vi "Force_command_IHS.vi"(11 "Data In":T1={"Core"={"Current VI Reference"=refnum, "Close Panel on Exit?"=FALSE, "Start Timestmap"="", "Status His"="", "Active"=FALSE, "Exit"=FALSE, "Assignment structure"=""}, "Sample ID"="", "Cam"={"Cam"="", "Connected"=FALSE, "Sim Image"=FALSE, "Save pictures"=FALSE}, "UR"={"PC_IP"="192.168.0.15", "Remote port"=30002, "UR_IP"="192.168.0.10", "connection ID"=refnum, "Connected"=FALSE, "Sim UR signal"=FALSE, "UR Ready"=FALSE, "Ready fail"=0.0}, "Sample data"={"Insects taken from current picture"=0, "Number of insects in pick-up area"=0, "Object data"={"Object CoM X"=0.0, "Object CoM Y"=0.0, "Corrected Object orientation"=0.0, "Object length"=0.0, "Z, Height"=0.0}, "Raw Particle Measurements"=[], "Insect-data-array"=[], "Sorted Particle Measurements"=[], "Insects to pick this round"=0, "Picking array"=[], "Pixels Measurements"=[], "Tool1 to pick"=0}, "Images"={"Image"=refnum, "Image Timestamp"="", "Boarder Image"=refnum, "Vision A. Image"=refnum}, "Reshake"=0, "Settings"={"Number to try and pick"=8, "Last few"=4, "Z_Zero"=0.0, "Tool switch size"=2.0, "X-Zero"=-35.0, "Y-Zero"=406.0, "Small or XL"=12.0, "Tool1-Height"=12.0, "Tool2-Height"=12.0, "Ignore small"=12.0, "Time to Whait"=25.0}, "Assignment"={"Executing Assignment"="", "Task"="", "Tool"="", "Specimen to pick"=0, "GO"=FALSE}, "Return reason"=""} {"Sample data"."Object data"."Z, Height" format="%#_13g"}) -> (1 "Command type":enum16{"Default", "Right", "Left"}(ring), 2 "Canceled":bool, 3 "Data Out":T1={"Core"={"Current VI Reference"=refnum, "Close Panel on Exit?"=FALSE, "Start Timestmap"="", "Status His"="", "Active"=FALSE, "Exit"=FALSE, "Assignment structure"=""}, "Sample ID"="", "Cam"={"Cam"="", "Connected"=FALSE, "Sim Image"=FALSE, "Save pictures"=FALSE}, "UR"={"PC_IP"="192.168.0.15", "Remote port"=30002, "UR_IP"="192.168.0.10", "connection ID"=refnum, "Connected"=FALSE, "Sim UR signal"=FALSE, "UR Ready"=FALSE, "Ready fail"=0.0}, "Sample data"={"Insects taken from current picture"=0, "Number of insects in pick-up area"=0, "Object data"={"Object CoM X"=0.0, "Object CoM Y"=0.0, "Corrected Object orientation"=0.0, "Object length"=0.0, "Z, Height"=0.0}, "Raw Particle Measurements"=[], "Insect-data-array"=[], "Sorted Particle Measurements"=[], "Insects to pick this round"=0, "Picking array"=[], "Pixels Measurements"=[], "Tool1 to pick"=0}, "Images"={"Image"=refnum, "Image Timestamp"="", "Boarder Image"=refnum, "Vision A. Image"=refnum}, "Reshake"=0, "Settings"={"Number to try and pick"=8, "Last few"=4, "Z_Zero"=0.1, "Tool switch size"=2.0, "X-Zero"=-35.0, "Y-Zero"=406.0, "Small or XL"=12.0, "Tool1-Height"=12.0, "Tool2-Height"=12.0, "Ignore small"=12.0, "Time to Whait"=25.0}, "Assignment"={"Executing Assignment"="", "Task"="", "Tool"="", "Specimen to pick"=0, "GO"=FALSE}, "Return reason"=""} {"Sample data"."Object data"."Z, Height" format="%#_13g"})   [LabVIEW 2024]
uses:
  SRS/controls/IHS_JKI.ctl
  <vilib>/userDefined/High Color/IMAQdx.ctl
  <vilib>/vision/Image Controls.llb/IMAQ Image.ctl
panel:
  in  "Left":T4
  in  "Right":cluster{"Specimen to pick":i32}
  out "Sample data.Insect-data-array":string[][](array[string])
  in  "Cancel Button":bool
  in  "OK Button":bool
  # "UR Task list:\n1 = take pic.\n2 = take pic. No light.\n3-6 = Shake.\n7 = Sample for Sta. Bio with Tool1.\n8 = Sample for Sta. Bio with Tool2.\n9 = Tool3.\n10 = Move with selected Tool to specified pos.\n14 = Sample for XL Bio. with Tool1.\n16 = Sample for XL Bio. with Tool2.\n55 = Reset UR"
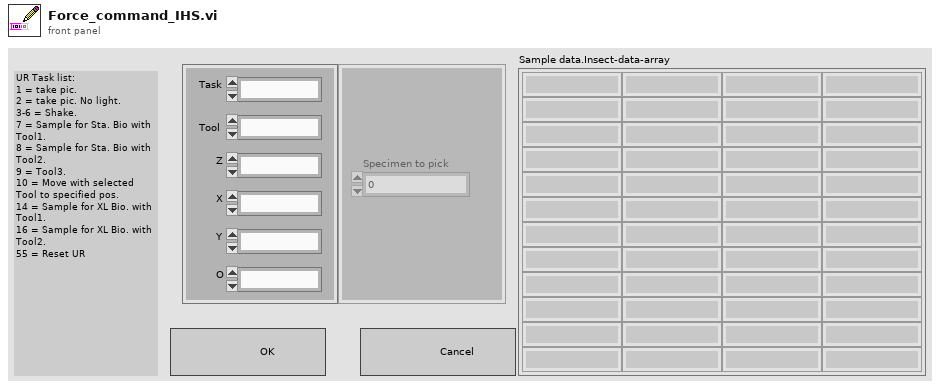
[diagram p1: front panel]
types:
  T1 = typedef "IHS_JKI.ctl" = cluster{"Core":cluster{"Current VI Reference":refnum<vi>, "Close Panel on Exit?":bool, "Start Timestmap":string, "Status His":string, "Active":bool, "Exit":bool, "Assignment structure":string}, "Sample ID":string, "Cam":cluster{"Cam":T2, "Connected":bool, "Sim Image":bool, "Save pictures":bool}, "UR":cluster{"PC_IP":string, "Remote port":u16, "UR_IP":string, "connection ID":refnum<k5>, "Connected":bool, "Sim UR signal":bool, "UR Ready":bool, "Ready fail":dbl}, "Sample data":cluster{"Insects taken from current picture":i32, "Number of insects in pick-up area":i32, "Object data":cluster{"Object CoM X":dbl, "Object CoM Y":dbl, "Corrected Object orientation":dbl, "Object length":dbl, "Z, Height":dbl}, "Raw Particle Measurements":dbl[][], "Insect-data-array":string[][], "Sorted Particle Measurements":dbl[][], "Insects to pick this round":i32, "Picking array":dbl[][], "Pixels Measurements":dbl[][], "Tool1 to pick":i32}, "Images":cluster{"Image":T3, "Image Timestamp":string, "Boarder Image":T3, "Vision A. Image":T3}, "Reshake":i32, "Settings":cluster{"Number to try and pick":i32, "Last few":i32, "Z_Zero":dbl, "Tool switch size":dbl, "X-Zero":dbl, "Y-Zero":dbl, "Small or XL":dbl, "Tool1-Height":dbl, "Tool2-Height":dbl, "Ignore small":dbl, "Time to Whait":dbl}, "Assignment":cluster{"Executing Assignment":string, "Task":string, "Tool":string, "Specimen to pick":i32, "GO":bool}, "Return reason":string}
  T2 = typedef "IMAQdx.ctl" = refnum<k21>
  T3 = typedef "IMAQ Image.ctl" = refnum<image>
  T4 = cluster{"Task":i32, "Tool":i32, "Y":dbl, "X":dbl, "Z":dbl, "O":dbl}
  T5 = enum8{"Enabled", "Disabled", "Disabled and Grayed Out"}
  T6 = cluster{"Number to try and pick":i32, "Last few":i32, "Z_Zero":dbl, "Tool switch size":dbl, "X-Zero":dbl, "Y-Zero":dbl, "Small or XL":dbl, "Tool1-Height":dbl, "Tool2-Height":dbl, "Ignore small":dbl, "Time to Whait":dbl}
  T7 = cluster{"Executing Assignment":string, "Task":string, "Tool":string, "Specimen to pick":i32, "GO":bool}
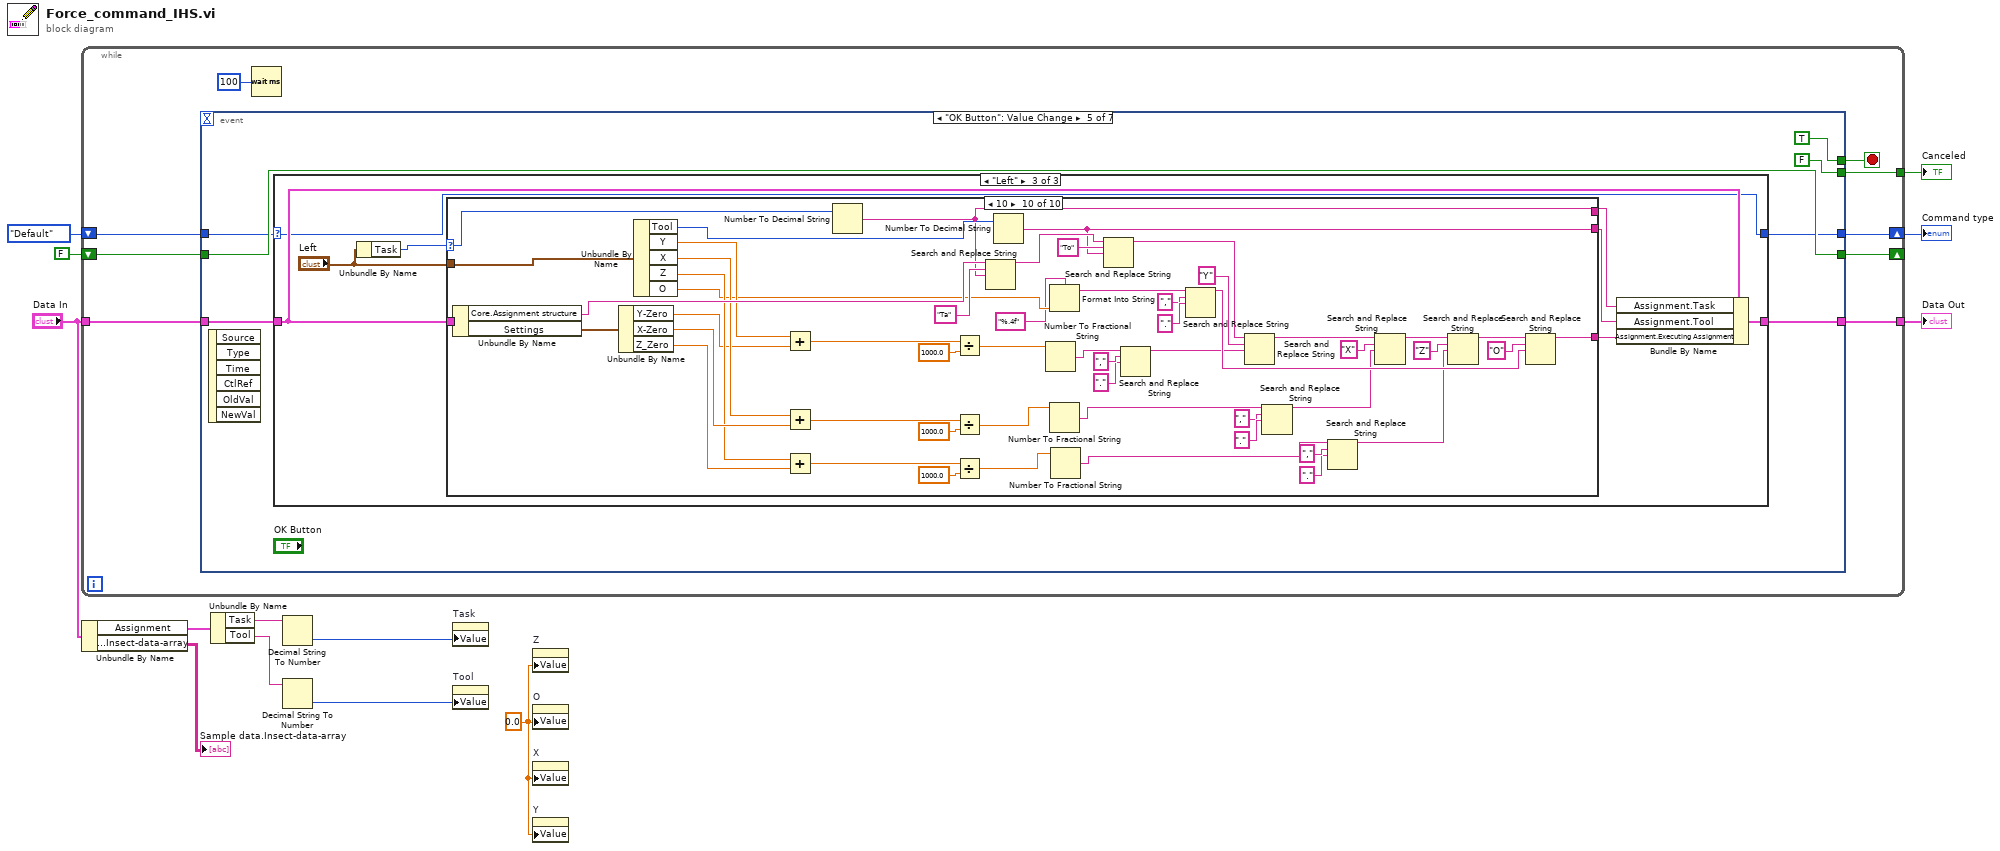
[diagram p0: block diagram]
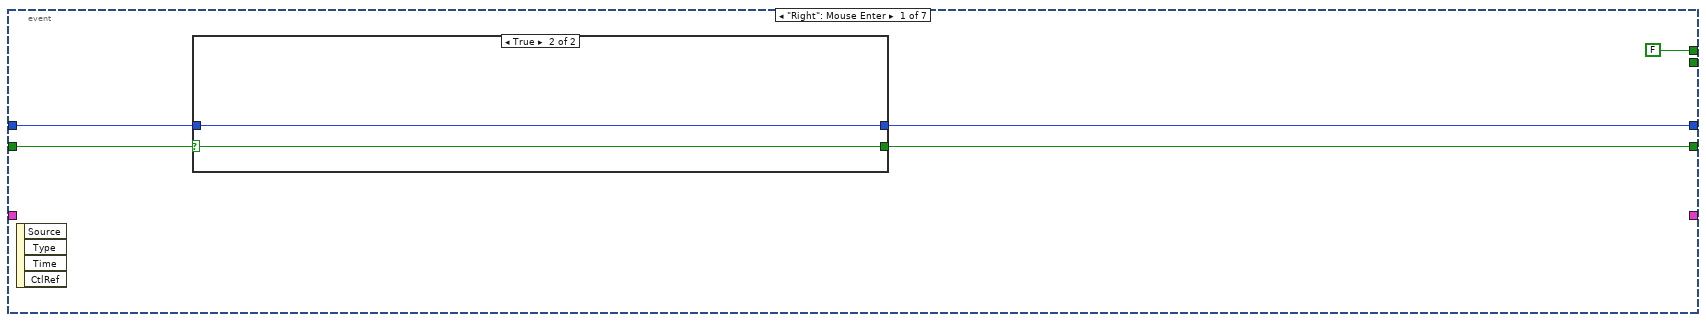
[diagram p2: hidden frame]
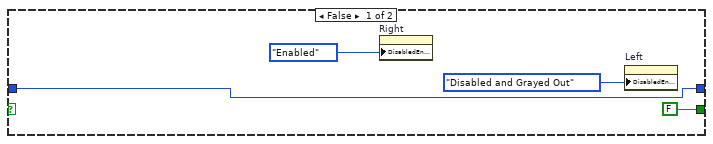
[diagram p3: hidden frame]
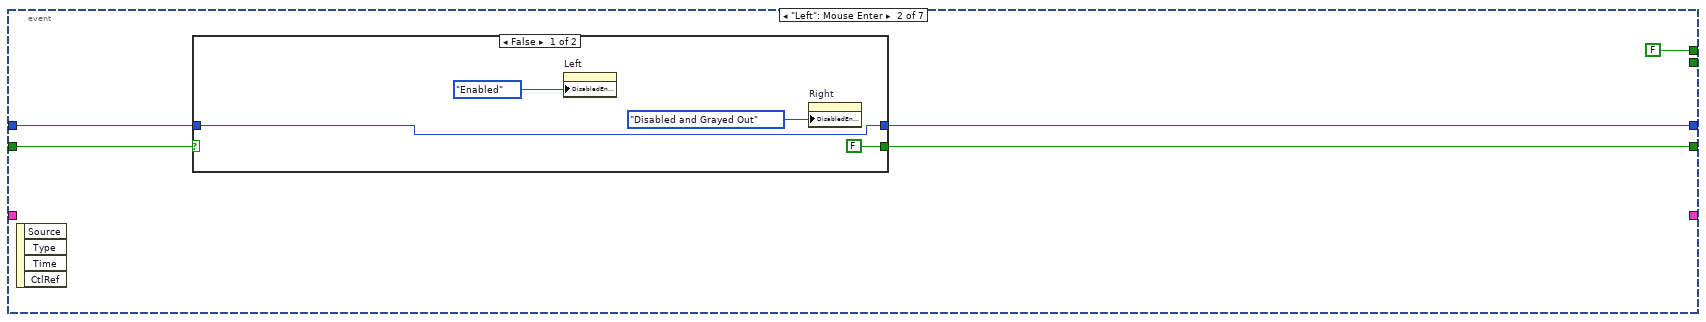
[diagram p4: hidden frame]
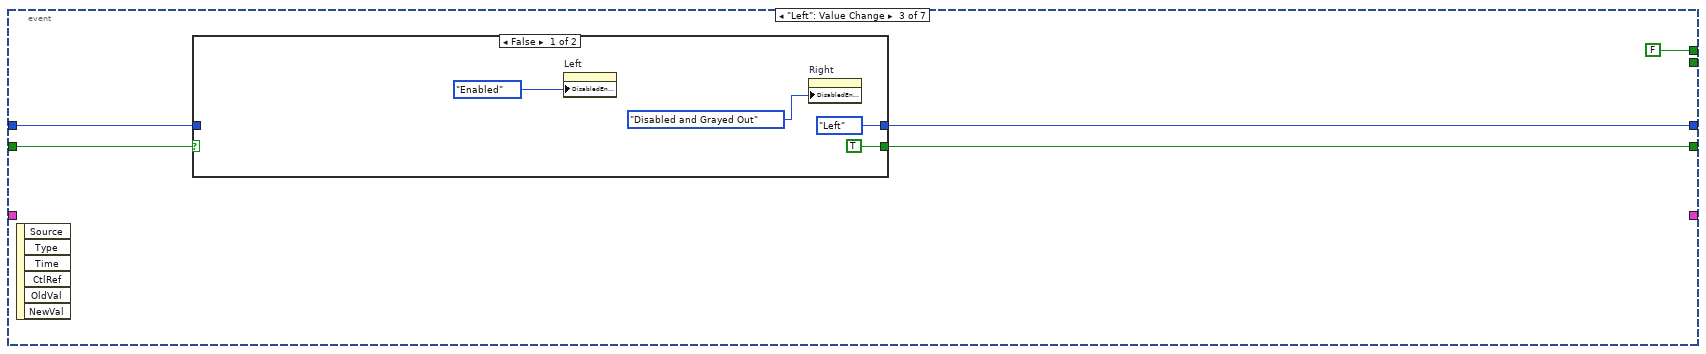
[diagram p6: hidden frame]
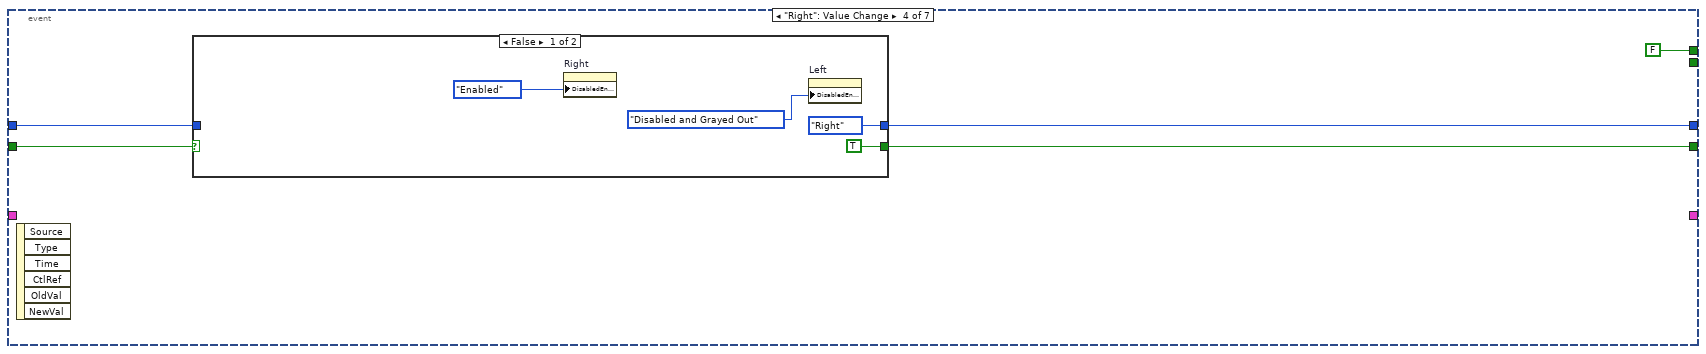
[diagram p8: hidden frame]
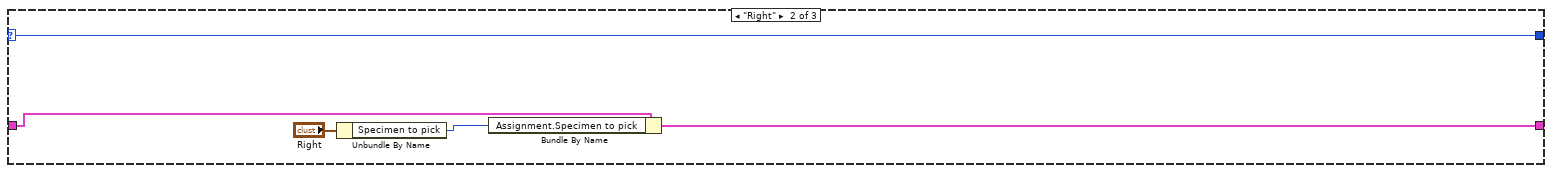
[diagram p11: hidden frame]
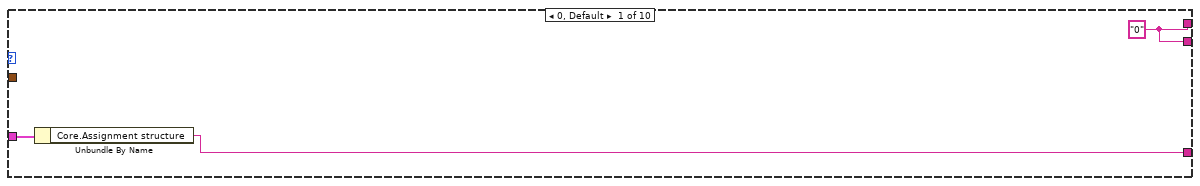
[diagram p12: hidden frame]
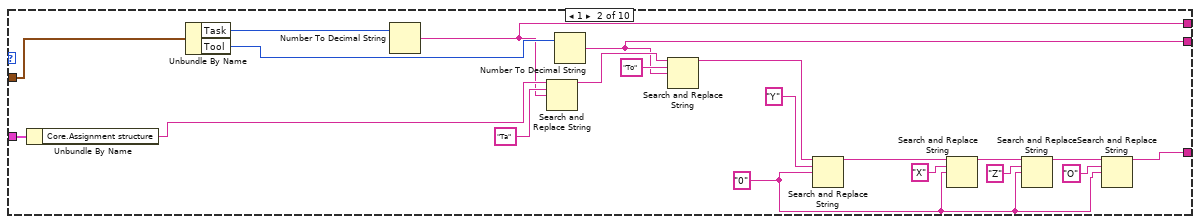
[diagram p13: hidden frame]
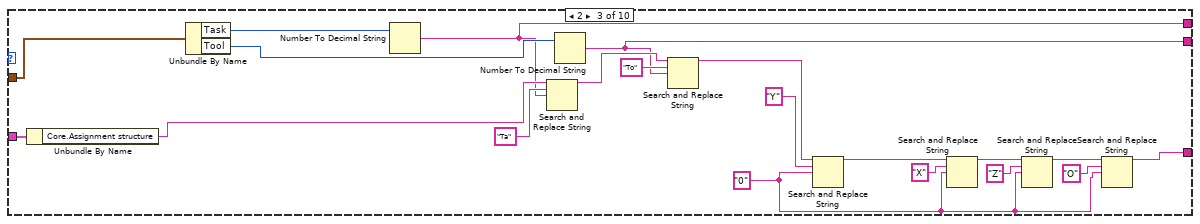
[diagram p14: hidden frame]
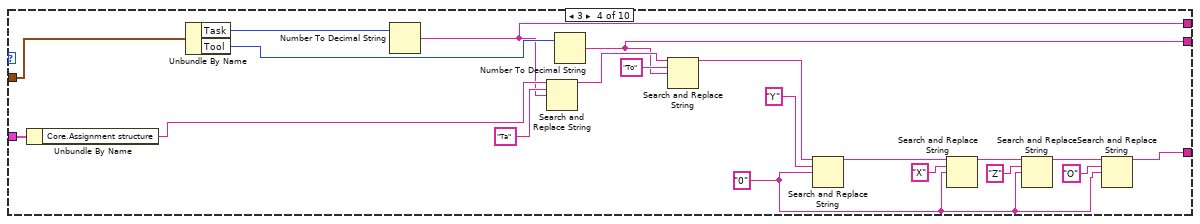
[diagram p15: hidden frame]
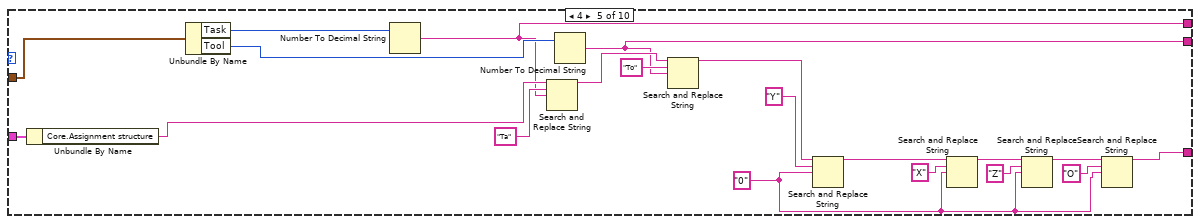
[diagram p16: hidden frame]
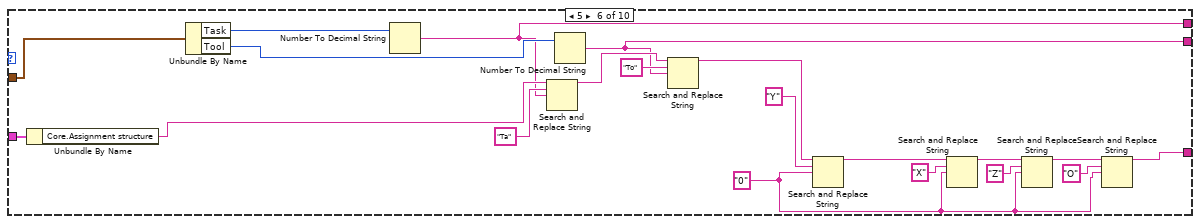
[diagram p17: hidden frame]
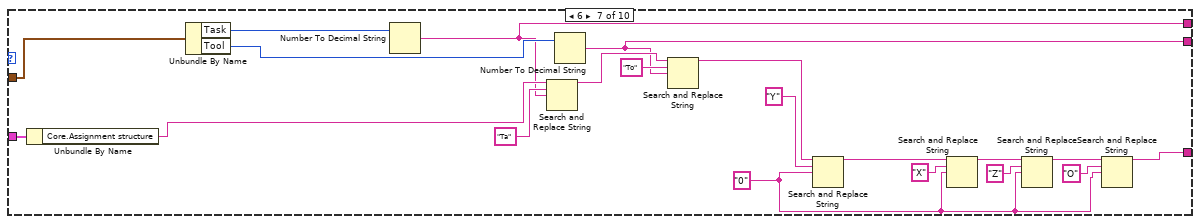
[diagram p18: hidden frame]
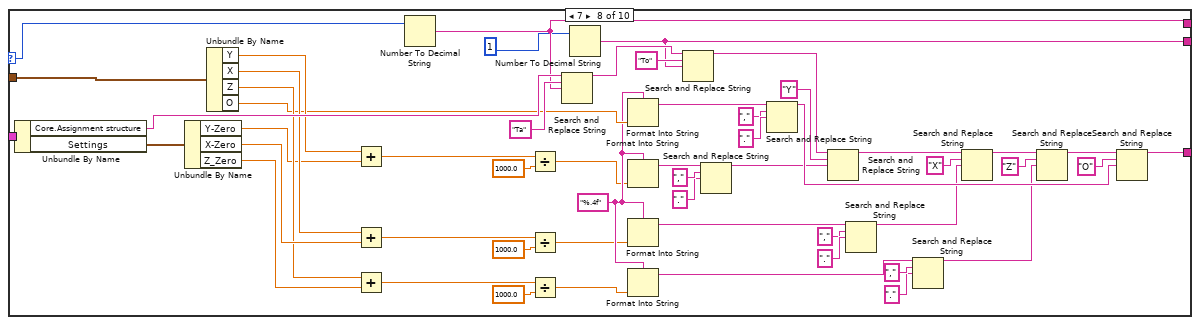
[diagram p19: hidden frame]
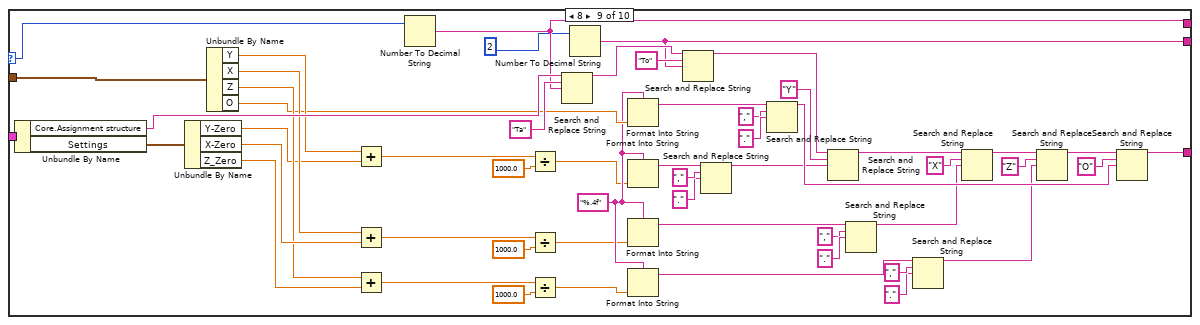
[diagram p20: hidden frame]
diagram:
  w1 = 0.0 ("Value")
  n1 = while {
    shift-right: [w20] -> _
    shift-left: FALSE -> [w21]
    shift-right: [w19] -> w5
    shift-left: enum16{"Default", "Right", "Left"}."Default" -> [w18]
    tunnel: "Data In" -> [w17]
    tunnel: [w16] -> w6
    tunnel: [w15] -> w4
    stop <- w14 stop-if-true
    n2 = event shown="[4] \"OK Button\": Value Change" {
      selector: _ -> [_ _ _ _ _ _ _]
      dyn-events: _ -> [_ _ _ _ _ _ _]
      timeout: _ -> [_ _ _ _ _ _ _]
      tunnel: [w27 w38 w47 w60 w72 w373 _] -> w20
      tunnel: [w26 w37 w49 w59 w68 enum16{"Default", "Right", "Left"}."Default" enum16{"Default", "Right", "Left"}."Default"] -> w19
      tunnel: w21 -> [w25 w36 w48 w58 w72 w373 _]
      tunnel: w18 -> [w24 w35 w46 w57 w69 _ _]
      tunnel: w17 -> [_ _ _ _ w73 w374 w378]
      tunnel: [_ _ _ _ FALSE TRUE TRUE] -> w16
      tunnel: [_ _ _ _ w70 w374 w378] -> w15
      tunnel: [FALSE FALSE FALSE FALSE TRUE TRUE TRUE] -> w14
      event "Right": Mouse Enter {
        n3 = event-data() -> ()  [unwired: 1 in, 4 out]
        n4 = case shown="True" w25 {
          selector: w25 -> [_ w33]
          tunnel: [FALSE w33] -> w27
          tunnel: [w28 w32] -> w26
          tunnel: w24 -> [w28 w32]
          frame False {
            n5 = property on="Right" class="Clust (strict)"("DisabledEnum"=T5."Enabled" ("Disabled")) -> ()  [unwired: 2 in, 2 out]
            n6 = property on="Left" class="Clust (strict)"("DisabledEnum"=T5."Disabled and Grayed Out" ("Disabled")) -> ()  [unwired: 2 in, 2 out]
          }
          frame True {
          }
        }
      }
      event "Left": Mouse Enter {
        n7 = event-data() -> ()  [unwired: 1 in, 4 out]
        n8 = case shown="False" w36 {
          selector: w36 -> [_ w44]
          tunnel: [FALSE w44] -> w38
          tunnel: [w39 w43] -> w37
          tunnel: w35 -> [w39 w43]
          frame False {
            n9 = property on="Left" class="Clust (strict)"("DisabledEnum"=T5."Enabled" ("Disabled")) -> ()  [unwired: 2 in, 2 out]
            n10 = property on="Right" class="Clust (strict)"("DisabledEnum"=T5."Disabled and Grayed Out" ("Disabled")) -> ()  [unwired: 2 in, 2 out]
          }
          frame True {
          }
        }
      }
      event "Left": Value Change {
        n11 = event-data() -> ()  [unwired: 1 in, 6 out]
        n12 = case shown="False" w48 {
          selector: w48 -> [_ w55]
          tunnel: [enum16{"Default", "Right", "Left"}."Left" w54] -> w49
          tunnel: [TRUE w55] -> w47
          tunnel: w46 -> [_ w54]
          frame False {
            n13 = property on="Left" class="Clust (strict)"("DisabledEnum"=T5."Enabled" ("Disabled")) -> ()  [unwired: 2 in, 2 out]
            n14 = property on="Right" class="Clust (strict)"("DisabledEnum"=T5."Disabled and Grayed Out" ("Disabled")) -> ()  [unwired: 2 in, 2 out]
          }
          frame True {
          }
        }
      }
      event "Right": Value Change {
        n15 = event-data() -> ()  [unwired: 1 in, 6 out]
        n16 = case shown="False" w58 {
          selector: w58 -> [_ w66]
          tunnel: [TRUE w66] -> w60
          tunnel: [enum16{"Default", "Right", "Left"}."Right" w65] -> w59
          tunnel: w57 -> [_ w65]
          frame False {
            n17 = property on="Right" class="Clust (strict)"("DisabledEnum"=T5."Enabled" ("Disabled")) -> ()  [unwired: 2 in, 2 out]
            n18 = property on="Left" class="Clust (strict)"("DisabledEnum"=T5."Disabled and Grayed Out" ("Disabled")) -> ()  [unwired: 2 in, 2 out]
          }
          frame True {
          }
        }
      }
      event "OK Button": Value Change {
        n19 = event-data() -> ()  [unwired: 1 in, 6 out]
        n20 = case shown="\"Left\"" w69 {
          selector: w69 -> [w74 w77 w84]
          tunnel: w73 -> [w75 w80 w88]
          tunnel: [w75 w79 w85] -> w70
          tunnel: [w74 w77 w84] -> w68
          frame "Default", Default {
          }
          frame "Right" {
            n21 = Unbundle By Name("Right") -> ("Specimen to pick"=w78:i32)
            n22 = Bundle By Name(cluster=w80, "Assignment.Specimen to pick"=w78) -> (w79:T1)
          }
          frame "Left" {
            n23 = Unbundle By Name("Left") -> ("Task"=w81:i32)
            n24 = case shown="10" w81 {
              selector: w81 -> [_ _ _ _ _ _ _ w214 w267 w325]
              tunnel: w88 -> [w91 w99 w119 w139 w159 w179 w199 w264 w317 w370]
              tunnel: [w89 w94 w114 w134 w154 w174 w194 w213 w266 w324] -> w87
              tunnel: [w89 w93 w113 w133 w153 w173 w193 w253 w306 w358] -> w86
              tunnel: "Left" -> [_ w97 w117 w137 w157 w177 w197 w252 w305 w357]
              tunnel: [w90 w95 w115 w135 w155 w175 w195 w243 w296 w348] -> w83
              frame 0, Default {
                w89 = "0"
                n25 = Unbundle By Name(w91) -> ("Core.Assignment structure"=w90:string)
              }
              frame 1 {
                w92 = "0" ("replace string (\"\")")
                n26 = Unbundle By Name(w99) -> ("Core.Assignment structure"=w98:string)
                n27 = Unbundle By Name(w97) -> ("Task"=w96:i32, "Tool"=w111:i32)
                n28 = Number To Decimal String(number=w96) -> (decimal integer string=w94:string)  [unwired: 1 in]
                n29 = Search and Replace String(input string=w98, search string="Ta", replace string=w94) -> (result string=w110:string)  [unwired: 5 in, 3 out]
                n30 = Number To Decimal String(number=w111) -> (decimal integer string=w93:string)  [unwired: 1 in]
                n31 = Search and Replace String(input string=w110, search string="To", replace string=w93) -> (result string=w109:string)  [unwired: 5 in, 3 out]
                n32 = Search and Replace String(input string=w109, search string="Y", replace string=w92) -> (result string=w108:string)  [unwired: 5 in, 3 out]
                n33 = Search and Replace String(input string=w108, search string="X", replace string=w92) -> (result string=w107:string)  [unwired: 5 in, 3 out]
                n34 = Search and Replace String(input string=w107, search string="Z", replace string=w92) -> (result string=w101:string)  [unwired: 5 in, 3 out]
                n35 = Search and Replace String(input string=w101, search string="O", replace string=w92) -> (result string=w95:string)  [unwired: 5 in, 3 out]
              }
              frame 2 {
                w112 = "0" ("replace string (\"\")")
                n36 = Unbundle By Name(w119) -> ("Core.Assignment structure"=w118:string)
                n37 = Unbundle By Name(w117) -> ("Task"=w116:i32, "Tool"=w131:i32)
                n38 = Number To Decimal String(number=w116) -> (decimal integer string=w114:string)  [unwired: 1 in]
                n39 = Search and Replace String(input string=w118, search string="Ta", replace string=w114) -> (result string=w130:string)  [unwired: 5 in, 3 out]
                n40 = Number To Decimal String(number=w131) -> (decimal integer string=w113:string)  [unwired: 1 in]
                n41 = Search and Replace String(input string=w130, search string="To", replace string=w113) -> (result string=w129:string)  [unwired: 5 in, 3 out]
                n42 = Search and Replace String(input string=w129, search string="Y", replace string=w112) -> (result string=w128:string)  [unwired: 5 in, 3 out]
                n43 = Search and Replace String(input string=w128, search string="X", replace string=w112) -> (result string=w127:string)  [unwired: 5 in, 3 out]
                n44 = Search and Replace String(input string=w127, search string="Z", replace string=w112) -> (result string=w121:string)  [unwired: 5 in, 3 out]
                n45 = Search and Replace String(input string=w121, search string="O", replace string=w112) -> (result string=w115:string)  [unwired: 5 in, 3 out]
              }
              frame 3 {
                w132 = "0" ("replace string (\"\")")
                n46 = Unbundle By Name(w139) -> ("Core.Assignment structure"=w138:string)
                n47 = Unbundle By Name(w137) -> ("Task"=w136:i32, "Tool"=w151:i32)
                n48 = Number To Decimal String(number=w136) -> (decimal integer string=w134:string)  [unwired: 1 in]
                n49 = Search and Replace String(input string=w138, search string="Ta", replace string=w134) -> (result string=w150:string)  [unwired: 5 in, 3 out]
                n50 = Number To Decimal String(number=w151) -> (decimal integer string=w133:string)  [unwired: 1 in]
                n51 = Search and Replace String(input string=w150, search string="To", replace string=w133) -> (result string=w149:string)  [unwired: 5 in, 3 out]
                n52 = Search and Replace String(input string=w149, search string="Y", replace string=w132) -> (result string=w148:string)  [unwired: 5 in, 3 out]
                n53 = Search and Replace String(input string=w148, search string="X", replace string=w132) -> (result string=w147:string)  [unwired: 5 in, 3 out]
                n54 = Search and Replace String(input string=w147, search string="Z", replace string=w132) -> (result string=w141:string)  [unwired: 5 in, 3 out]
                n55 = Search and Replace String(input string=w141, search string="O", replace string=w132) -> (result string=w135:string)  [unwired: 5 in, 3 out]
              }
              frame 4 {
                w152 = "0" ("replace string (\"\")")
                n56 = Unbundle By Name(w159) -> ("Core.Assignment structure"=w158:string)
                n57 = Unbundle By Name(w157) -> ("Task"=w156:i32, "Tool"=w171:i32)
                n58 = Number To Decimal String(number=w156) -> (decimal integer string=w154:string)  [unwired: 1 in]
                n59 = Search and Replace String(input string=w158, search string="Ta", replace string=w154) -> (result string=w170:string)  [unwired: 5 in, 3 out]
                n60 = Number To Decimal String(number=w171) -> (decimal integer string=w153:string)  [unwired: 1 in]
                n61 = Search and Replace String(input string=w170, search string="To", replace string=w153) -> (result string=w169:string)  [unwired: 5 in, 3 out]
                n62 = Search and Replace String(input string=w169, search string="Y", replace string=w152) -> (result string=w168:string)  [unwired: 5 in, 3 out]
                n63 = Search and Replace String(input string=w168, search string="X", replace string=w152) -> (result string=w167:string)  [unwired: 5 in, 3 out]
                n64 = Search and Replace String(input string=w167, search string="Z", replace string=w152) -> (result string=w161:string)  [unwired: 5 in, 3 out]
                n65 = Search and Replace String(input string=w161, search string="O", replace string=w152) -> (result string=w155:string)  [unwired: 5 in, 3 out]
              }
              frame 5 {
                w172 = "0" ("replace string (\"\")")
                n66 = Unbundle By Name(w179) -> ("Core.Assignment structure"=w178:string)
                n67 = Unbundle By Name(w177) -> ("Task"=w176:i32, "Tool"=w191:i32)
                n68 = Number To Decimal String(number=w176) -> (decimal integer string=w174:string)  [unwired: 1 in]
                n69 = Search and Replace String(input string=w178, search string="Ta", replace string=w174) -> (result string=w190:string)  [unwired: 5 in, 3 out]
                n70 = Number To Decimal String(number=w191) -> (decimal integer string=w173:string)  [unwired: 1 in]
                n71 = Search and Replace String(input string=w190, search string="To", replace string=w173) -> (result string=w189:string)  [unwired: 5 in, 3 out]
                n72 = Search and Replace String(input string=w189, search string="Y", replace string=w172) -> (result string=w188:string)  [unwired: 5 in, 3 out]
                n73 = Search and Replace String(input string=w188, search string="X", replace string=w172) -> (result string=w187:string)  [unwired: 5 in, 3 out]
                n74 = Search and Replace String(input string=w187, search string="Z", replace string=w172) -> (result string=w181:string)  [unwired: 5 in, 3 out]
                n75 = Search and Replace String(input string=w181, search string="O", replace string=w172) -> (result string=w175:string)  [unwired: 5 in, 3 out]
              }
              frame 6 {
                w192 = "0" ("replace string (\"\")")
                n76 = Unbundle By Name(w199) -> ("Core.Assignment structure"=w198:string)
                n77 = Unbundle By Name(w197) -> ("Task"=w196:i32, "Tool"=w211:i32)
                n78 = Number To Decimal String(number=w196) -> (decimal integer string=w194:string)  [unwired: 1 in]
                n79 = Search and Replace String(input string=w198, search string="Ta", replace string=w194) -> (result string=w210:string)  [unwired: 5 in, 3 out]
                n80 = Number To Decimal String(number=w211) -> (decimal integer string=w193:string)  [unwired: 1 in]
                n81 = Search and Replace String(input string=w210, search string="To", replace string=w193) -> (result string=w209:string)  [unwired: 5 in, 3 out]
                n82 = Search and Replace String(input string=w209, search string="Y", replace string=w192) -> (result string=w208:string)  [unwired: 5 in, 3 out]
                n83 = Search and Replace String(input string=w208, search string="X", replace string=w192) -> (result string=w207:string)  [unwired: 5 in, 3 out]
                n84 = Search and Replace String(input string=w207, search string="Z", replace string=w192) -> (result string=w201:string)  [unwired: 5 in, 3 out]
                n85 = Search and Replace String(input string=w201, search string="O", replace string=w192) -> (result string=w195:string)  [unwired: 5 in, 3 out]
              }
              frame 7 {
                w226 = "%.4f" ("format string")
                n86 = Unbundle By Name(w264) -> ("Core.Assignment structure"=w263:string, "Settings"=w251:T6)
                n87 = Unbundle By Name(w251) -> ("Y-Zero"=w245:dbl, "X-Zero"=w248:dbl, "Z_Zero"=w246:dbl)
                n88 = Unbundle By Name(w252) -> ("Y"=w250:dbl, "X"=w249:dbl, "Z"=w247:dbl, "O"=w241:dbl)
                n89 = Add(x=w250, y=w245) -> (x+y=w223:dbl)
                n90 = Add(x=w249, y=w248) -> (x+y=w219:dbl)
                n91 = Add(x=w247, y=w246) -> (x+y=w215:dbl)
                n92 = Number To Decimal String(number=w214) -> (decimal integer string=w213:string)  [unwired: 1 in]
                n93 = Divide(x=w223, y=1000.0) -> (x/y=w224:dbl)
                n94 = Divide(x=w219, y=1000.0) -> (x/y=w220:dbl)
                n95 = Divide(x=w215, y=1000.0) -> (x/y=w216:dbl)
                n96 = Search and Replace String(input string=w263, search string="Ta", replace string=w213) -> (result string=w262:string)  [unwired: 5 in, 3 out]
                n97 = Number To Decimal String(number=1) -> (decimal integer string=w253:string)  [unwired: 1 in]
                n98 = Format Into String(format string=w226, w241) -> (resulting string=w231:string)  [unwired: 2 in, 1 out]
                n99 = Format Into String(format string=w226, w224) -> (resulting string=w240:string)  [unwired: 2 in, 1 out]
                n100 = Format Into String(format string=w226, w220) -> (resulting string=w221:string)  [unwired: 2 in, 1 out]
                n101 = Format Into String(format string=w226, w216) -> (resulting string=w228:string)  [unwired: 2 in, 1 out]
                n102 = Search and Replace String(input string=w262, search string="To", replace string=w253) -> (result string=w261:string)  [unwired: 5 in, 3 out]
                n103 = Search and Replace String(input string=w240, search string=",", replace string="." ("replace string (\"\")")) -> (result string=w222:string)  [unwired: 5 in, 3 out]
                n104 = Search and Replace String(input string=w231, search string=",", replace string="." ("replace string (\"\")")) -> (result string=w230:string)  [unwired: 5 in, 3 out]
                n105 = Search and Replace String(input string=w261, search string="Y", replace string=w222) -> (result string=w260:string)  [unwired: 5 in, 3 out]
                n106 = Search and Replace String(input string=w221, search string=",", replace string="." ("replace string (\"\")")) -> (result string=w227:string)  [unwired: 5 in, 3 out]
                n107 = Search and Replace String(input string=w228, search string=",", replace string="." ("replace string (\"\")")) -> (result string=w229:string)  [unwired: 5 in, 3 out]
                n108 = Search and Replace String(input string=w260, search string="X", replace string=w227) -> (result string=w259:string)  [unwired: 5 in, 3 out]
                n109 = Search and Replace String(input string=w259, search string="Z", replace string=w229) -> (result string=w244:string)  [unwired: 5 in, 3 out]
                n110 = Search and Replace String(input string=w244, search string="O", replace string=w230) -> (result string=w243:string)  [unwired: 5 in, 3 out]
              }
              frame 8 {
                w279 = "%.4f" ("format string")
                n111 = Unbundle By Name(w317) -> ("Core.Assignment structure"=w316:string, "Settings"=w304:T6)
                n112 = Unbundle By Name(w304) -> ("Y-Zero"=w298:dbl, "X-Zero"=w301:dbl, "Z_Zero"=w299:dbl)
                n113 = Unbundle By Name(w305) -> ("Y"=w303:dbl, "X"=w302:dbl, "Z"=w300:dbl, "O"=w294:dbl)
                n114 = Add(x=w303, y=w298) -> (x+y=w276:dbl)
                n115 = Add(x=w302, y=w301) -> (x+y=w272:dbl)
                n116 = Add(x=w300, y=w299) -> (x+y=w268:dbl)
                n117 = Number To Decimal String(number=w267) -> (decimal integer string=w266:string)  [unwired: 1 in]
                n118 = Divide(x=w276, y=1000.0) -> (x/y=w277:dbl)
                n119 = Divide(x=w272, y=1000.0) -> (x/y=w273:dbl)
                n120 = Divide(x=w268, y=1000.0) -> (x/y=w269:dbl)
                n121 = Search and Replace String(input string=w316, search string="Ta", replace string=w266) -> (result string=w315:string)  [unwired: 5 in, 3 out]
                n122 = Number To Decimal String(number=2) -> (decimal integer string=w306:string)  [unwired: 1 in]
                n123 = Format Into String(format string=w279, w294) -> (resulting string=w284:string)  [unwired: 2 in, 1 out]
                n124 = Format Into String(format string=w279, w277) -> (resulting string=w293:string)  [unwired: 2 in, 1 out]
                n125 = Format Into String(format string=w279, w273) -> (resulting string=w274:string)  [unwired: 2 in, 1 out]
                n126 = Format Into String(format string=w279, w269) -> (resulting string=w281:string)  [unwired: 2 in, 1 out]
                n127 = Search and Replace String(input string=w315, search string="To", replace string=w306) -> (result string=w314:string)  [unwired: 5 in, 3 out]
                n128 = Search and Replace String(input string=w293, search string=",", replace string="." ("replace string (\"\")")) -> (result string=w275:string)  [unwired: 5 in, 3 out]
                n129 = Search and Replace String(input string=w284, search string=",", replace string="." ("replace string (\"\")")) -> (result string=w283:string)  [unwired: 5 in, 3 out]
                n130 = Search and Replace String(input string=w314, search string="Y", replace string=w275) -> (result string=w313:string)  [unwired: 5 in, 3 out]
                n131 = Search and Replace String(input string=w274, search string=",", replace string="." ("replace string (\"\")")) -> (result string=w280:string)  [unwired: 5 in, 3 out]
                n132 = Search and Replace String(input string=w281, search string=",", replace string="." ("replace string (\"\")")) -> (result string=w282:string)  [unwired: 5 in, 3 out]
                n133 = Search and Replace String(input string=w313, search string="X", replace string=w280) -> (result string=w312:string)  [unwired: 5 in, 3 out]
                n134 = Search and Replace String(input string=w312, search string="Z", replace string=w282) -> (result string=w297:string)  [unwired: 5 in, 3 out]
                n135 = Search and Replace String(input string=w297, search string="O", replace string=w283) -> (result string=w296:string)  [unwired: 5 in, 3 out]
              }
              frame 10 {
                n136 = Unbundle By Name(w370) -> ("Core.Assignment structure"=w368:string, "Settings"=w356:T6)
                n137 = Unbundle By Name(w356) -> ("Y-Zero"=w350:dbl, "X-Zero"=w353:dbl, "Z_Zero"=w351:dbl)
                n138 = Unbundle By Name(w357) -> ("Tool"=w369:i32, "Y"=w355:dbl, "X"=w354:dbl, "Z"=w352:dbl, "O"=w346:dbl)
                n139 = Add(x=w355, y=w350) -> (x+y=w331:dbl)
                n140 = Add(x=w354, y=w353) -> (x+y=w329:dbl)
                n141 = Add(x=w352, y=w351) -> (x+y=w326:dbl)
                n142 = Number To Decimal String(number=w325) -> (decimal integer string=w324:string)  [unwired: 1 in]
                n143 = Divide(x=w331, y=1000.0) -> (x/y=w322:dbl)
                n144 = Divide(x=w329, y=1000.0) -> (x/y=w318:dbl)
                n145 = Divide(x=w326, y=1000.0) -> (x/y=w319:dbl)
                n146 = Search and Replace String(input string=w368, search string="Ta", replace string=w324) -> (result string=w367:string)  [unwired: 5 in, 3 out]
                n147 = Number To Decimal String(number=w369) -> (decimal integer string=w358:string)  [unwired: 1 in]
                n148 = Number To Fractional String(number=w322) -> (F-format string=w323:string)  [unwired: 3 in]
                n149 = Format Into String(format string="%.4f", w346) -> (resulting string=w337:string)  [unwired: 2 in, 1 out]
                n150 = Number To Fractional String(number=w318) -> (F-format string=w321:string)  [unwired: 3 in]
                n151 = Number To Fractional String(number=w319) -> (F-format string=w320:string)  [unwired: 3 in]
                n152 = Search and Replace String(input string=w367, search string="To", replace string=w358) -> (result string=w366:string)  [unwired: 5 in, 3 out]
                n153 = Search and Replace String(input string=w323, search string=",", replace string="." ("replace string (\"\")")) -> (result string=w330:string)  [unwired: 5 in, 3 out]
                n154 = Search and Replace String(input string=w337, search string=",", replace string="." ("replace string (\"\")")) -> (result string=w336:string)  [unwired: 5 in, 3 out]
                n155 = Search and Replace String(input string=w366, search string="Y", replace string=w330) -> (result string=w365:string)  [unwired: 5 in, 3 out]
                n156 = Search and Replace String(input string=w321, search string=",", replace string="." ("replace string (\"\")")) -> (result string=w334:string)  [unwired: 5 in, 3 out]
                n157 = Search and Replace String(input string=w320, search string=",", replace string="." ("replace string (\"\")")) -> (result string=w335:string)  [unwired: 5 in, 3 out]
                n158 = Search and Replace String(input string=w365, search string="X", replace string=w334) -> (result string=w364:string)  [unwired: 5 in, 3 out]
                n159 = Search and Replace String(input string=w364, search string="Z", replace string=w335) -> (result string=w349:string)  [unwired: 5 in, 3 out]
                n160 = Search and Replace String(input string=w349, search string="O", replace string=w336) -> (result string=w348:string)  [unwired: 5 in, 3 out]
              }
            }
            n161 = Bundle By Name(cluster=w88, "Assignment.Task"=w87, "Assignment.Tool"=w86, "Assignment.Executing Assignment"=w83) -> (w85:T1)
          }
        }
      }
      event "Cancel Button": Value Change {
        n162 = event-data() -> ()  [unwired: 1 in, 6 out]
      }
      event Panel Close {
        n163 = event-data() -> ()  [unwired: 1 in, 4 out]
      }
    }
    n164 = Wait (ms)(milliseconds to wait=u32 100) -> ()  [unwired: 1 out]
  }
  "Data Out" <- w4
  "Command type" <- w5
  "Canceled" <- w6
  n165 = Unbundle By Name("Data In") -> ("Assignment"=w13:T7, "Sample data.Insect-data-array"=→"Sample data.Insect-data-array":string[][])
  n166 = Unbundle By Name(w13) -> ("Task"=w11:string, "Tool"=w10:string)
  n167 = Decimal String To Number(string=w11) -> (number=w3:i32)  [unwired: 2 in, 1 out]
  n168 = Decimal String To Number(string=w10) -> (number=w2:i32)  [unwired: 2 in, 1 out]
  n169 = property on="Task" class="DigNum (strict)"("Value"=w3) -> ()  [unwired: 2 in, 2 out]
  n170 = property on="Tool" class="DigNum (strict)"("Value"=w2) -> ()  [unwired: 2 in, 2 out]
  n171 = property on="Z" class="DigNum (strict)"("Value"=w1) -> ()  [unwired: 2 in, 2 out]
  n172 = property on="O" class="DigNum (strict)"("Value"=w1) -> ()  [unwired: 2 in, 2 out]
  n173 = property on="X" class="DigNum (strict)"("Value"=w1) -> ()  [unwired: 2 in, 2 out]
  n174 = property on="Y" class="DigNum (strict)"("Value"=w1) -> ()  [unwired: 2 in, 2 out]
